vi "fileSelect.vi"() -> ()   [LabVIEW 2012]
panel:
  in  "Enter File Path":path
  out "File Path":path
  in  "File Comments":string
  in  "File Name":string caption="Beginning Text"
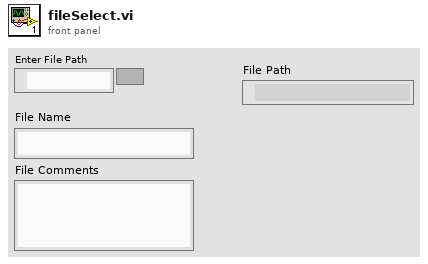
[diagram p1: front panel]
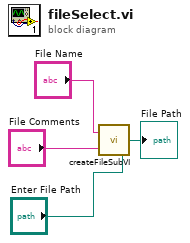
[diagram p0: block diagram]
diagram:
  n1 = call "createFileSubVI.vi"("File Name"="File Name", "File Comments"="File Comments", "Path For File"="Enter File Path") -> ("File Path"=→"File Path":path)  [unwired: 1 out]
